vi "ReadOutTiffPicture_v3.vi"(4 "Check Overexposure":bool, 5 "Binning size":i32, 6 "Overexposure threshold":dbl, 7 "Path":path=path "\\\\Walnuss\\Silverbrick/Lab/Stefan/Data/041108/C63/s_0001.b16") -> (0 "Overexposure?":bool, 1 "Height":i32, 2 "Width":i32, 3 "Indicator":dbl[][](array[numeric]))   [LabVIEW 2010]
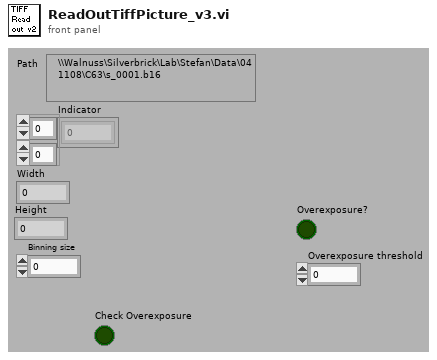
[diagram p1: front panel]
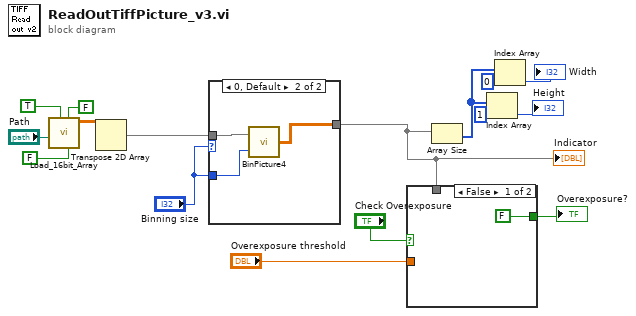
[diagram p0: block diagram]
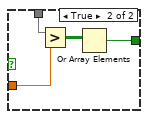
[diagram p2: hidden frame]
diagram:
  n1 = call "Load_16bit_Array.vi"("Load in PCO Format"=FALSE, "Load Array"=FALSE, "Take Full Path"=TRUE, "Path"="Path") -> ("Fluorescence Image"=w15:dbl[][])  [unwired: 6 in, 1 out]
  n2 = Transpose 2D Array(2D array=w15) -> (transposed array=w6:dbl[][])
  n3 = case shown="0, Default" "Binning size" {
    tunnel: w6 -> [w17 w20]
    tunnel: [w17 w19] -> w5
    tunnel: "Binning size" -> [_ w18]
    frame 1 {
    }
    frame 0, Default {
      n4 = call "BinPicture4.vi"("Binning size"=w18, "To bin"=w20) -> ("Output"=w19:dbl[][])
    }
  }
  "Indicator" <- w5
  n5 = case shown="False" "Check Overexposure" {
    tunnel: w5 -> [_ w25]
    tunnel: "Overexposure threshold" -> [_ w24]
    tunnel: [FALSE w22] -> w3
    frame False {
    }
    frame True {
      n6 = Greater?(x=w25, y=w24) -> (0:w23:bool[][])
      n7 = Or Array Elements(Boolean array=w23) -> (logical OR=w22:bool)
    }
  }
  "Overexposure?" <- w3
  n8 = Array Size(array=w5) -> (size(s)=w12:i32[])
  n9 = Index Array(array=w12, index=1) -> (element=→"Height":i32)
  n10 = Index Array(array=w12, index=0) -> (element=→"Width":i32)
